vi "Boolean (2D) to U8 (1D).vi"(0 "Bits":i32[](array[numeric]), 7 "Data":bool[][](array[boolean])) -> (8 "sum":u8[](array[numeric]))   [LabVIEW 2020]
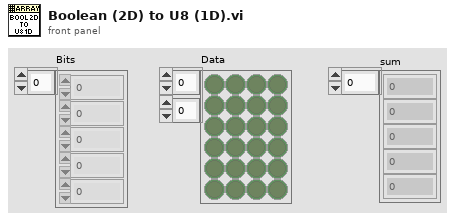
[diagram p1: front panel]
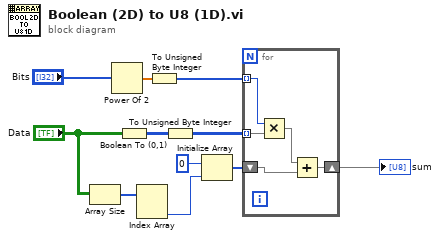
[diagram p0: block diagram]
diagram:
  n1 = Array Size(array="Data") -> (size(s)=w5:i32[])
  n2 = Power Of 2(x="Bits") -> (2^x=w11:dbl[])
  n3 = Boolean To (0,1)(Boolean="Data") -> (0, 1=w9:i16[][])
  n4 = Index Array(array=w5) -> (element #2=w4:i32)  [unwired: 2 in, 1 out]
  n5 = To Unsigned Byte Integer(number=w11) -> (unsigned 8bit integer=w8:u8[])
  n6 = To Unsigned Byte Integer(number=w9) -> (unsigned 8bit integer=w1:u8[][])
  n7 = Initialize Array(u8 0, w4) -> (w3:u8[])
  n8 = for {
    tunnel: w1 -> [w16] mode=indexing
    tunnel: w8 -> [w15] mode=indexing
    shift-right: [w12] -> w2
    shift-left: w3 -> [w14]
    n9 = Multiply(x=w15, y=w16) -> (x*y=w13:u8[])
    n10 = Add(x=w13, y=w14) -> (x+y=w12:u8[])
  }
  "sum" <- w2
